vi "P1dB_Anritsu_SA.vi"(0 "VISA resource name":refnum<visa-resource-name>, 5 "Marker (10:Active Marker)":i32(ring)=10 items=["Marker 1", "Marker 2", "Marker 3", "Marker 4", "Marker 5", "Marker 6", "Marker 7", "Marker 8", "Marker 9", "Marker 10", "Active Marker"], 7 "Marker Type (0:Frequency or Time)":i32(ring) items=["Frequency or Time", "Level", "Position"], 11 "error in (no error)":errorcluster) -> (4 "VISA resource name out":refnum<visa-resource-name>, 6 "Marker_X Response":dbl format="%.3f", 10 "Marker_Y Response 2":dbl format="%.3f", 15 "error out":errorcluster)   [LabVIEW 2020]
doc: "Reads the active Marker data."
uses:
  Anritsu Signal Analyzer Series/Anritsu Signal Analyzer Series.lvlib
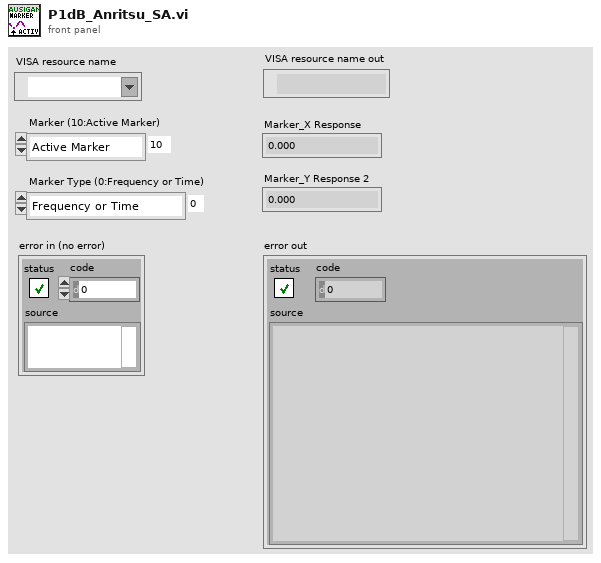
[diagram p1: front panel]
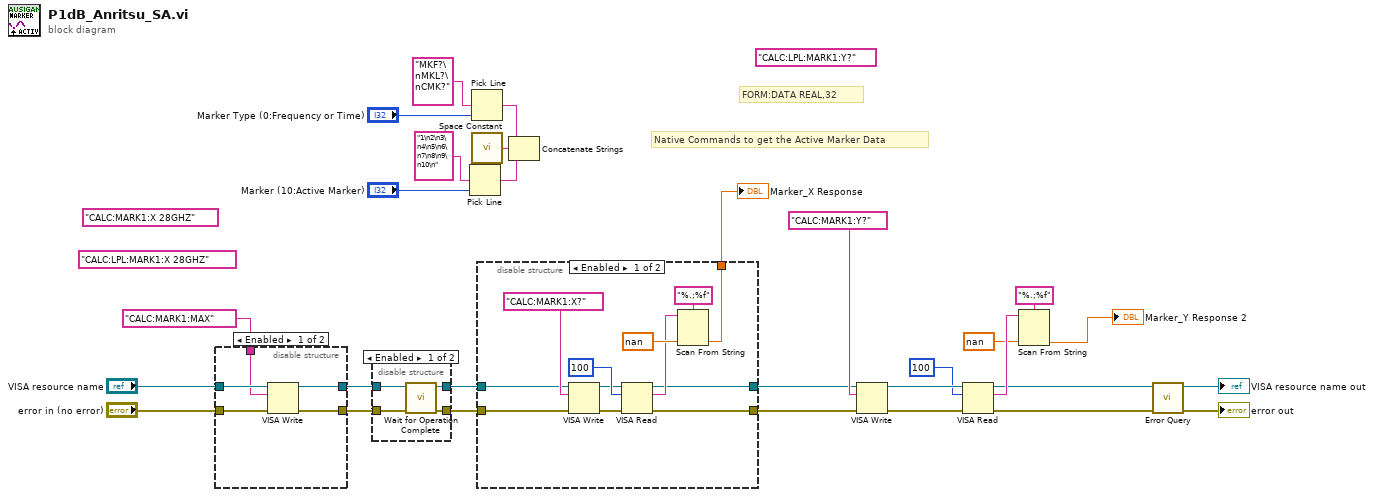
[diagram p0: block diagram]
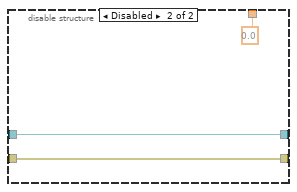
[diagram p2: hidden frame]
diagram:
  (unwired) "CALC:LPL:MARK1:Y?" ("write buffer")
  (unwired) "CALC:LPL:MARK1:X 28GHZ" ("write buffer")
  (unwired) "CALC:MARK1:X 28GHZ" ("write buffer")
  # "FORM:DATA REAL,32"
  # "Native Commands to get the Active Marker Data"
  n1 = disable-structure shown="Enabled" {
    disable-tunnel: "error in (no error)" -> [w34 w35]
    disable-tunnel: "VISA resource name" -> [w33 w36]
    disable-tunnel: [w32 w35] -> w17
    disable-tunnel: [w31 w36] -> w15
    disable-tunnel: "CALC:MARK1:MAX" ("write buffer") -> [w30 _]
    frame Enabled {
      n2 = VISA Write(VISA resource name=w33, write buffer=w30, error in (no error)=w34) -> (VISA resource name out=w31:refnum<visa-resource-name>, error out=w32:errorcluster)  [unwired: 1 out]
    }
    frame Disabled {
    }
  }
  n3 = disable-structure shown="Enabled" {
    disable-tunnel: w17 -> [w40 w41]
    disable-tunnel: [w39 w41] -> w16
    disable-tunnel: w15 -> [w38 w42]
    disable-tunnel: [w37 w42] -> w14
    frame Enabled {
      n4 = call "Wait for Operation Complete.vi"("error in (no error)"=w40, "VISA resource name"=w38) -> ("error out"=w39:errorcluster, "VISA resource name out"=w37:refnum<visa-resource-name>)  [unwired: 8 in]
    }
    frame Disabled {
    }
  }
  n5 = Pick Line(multi-line string="1\n2\n3\n4\n5\n6\n7\n8\n9\n10\n" ("文字列"), line index="Marker (10:Active Marker)") -> (output string=w24:string)  [unwired: 1 in]
  n6 = Pick Line(multi-line string="MKF?\nMKL?\nCMK?" ("_Command"), line index="Marker Type (0:Frequency or Time)") -> (output string=w20:string)  [unwired: 1 in]
  n7 = call <vilib>:"Space Constant.vi"() -> ("String"=w21:string)
  n8 = disable-structure shown="Enabled" {
    disable-tunnel: [w54 0.0 ("Marker_X Response")] -> w27
    disable-tunnel: w16 -> [w46 w56]
    disable-tunnel: w14 -> [w45 w57]
    disable-tunnel: [w44 w57] -> w2
    disable-tunnel: [w43 w56] -> w1
    frame Enabled {
      n9 = VISA Write(VISA resource name=w45, write buffer="CALC:MARK1:X?", error in (no error)=w46) -> (VISA resource name out=w48:refnum<visa-resource-name>, error out=w49:errorcluster)  [unwired: 1 out]
      n10 = VISA Read(VISA resource name=w48, byte count=u32 100 ("byte count (0)"), error in (no error)=w49) -> (VISA resource name out=w44:refnum<visa-resource-name>, read buffer=w51:string, error out=w43:errorcluster)  [unwired: 1 out]
      n11 = Scan From String(format string="%.;%f" ("Format String"), input string=w51, default 1=nan ("_Default")) -> (output 1=w54:dbl)  [unwired: 2 in, 3 out]
    }
    frame Disabled {
    }
  }
  "Marker_X Response" <- w27
  n12 = Concatenate Strings(w20, w21, w24) -> ()  [unwired: 1 out]
  n13 = VISA Write(VISA resource name=w2, write buffer="CALC:MARK1:Y?", error in (no error)=w1) -> (VISA resource name out=w12:refnum<visa-resource-name>, error out=w11:errorcluster)  [unwired: 1 out]
  n14 = VISA Read(VISA resource name=w12, byte count=u32 100 ("byte count (0)"), error in (no error)=w11) -> (VISA resource name out=w6:refnum<visa-resource-name>, read buffer=w9:string, error out=w5:errorcluster)  [unwired: 1 out]
  n15 = Scan From String(format string="%.;%f" ("Format String"), input string=w9, default 1=nan ("_Default")) -> (output 1=→"Marker_Y Response 2":dbl)  [unwired: 2 in, 3 out]
  n16 = call "Error Query.vi"("error in (no error)"=w5, "VISA resource name"=w6) -> ("error out"=→"error out":errorcluster, "VISA resource name out"=→"VISA resource name out":refnum<visa-resource-name>)  [unwired: 6 in, 2 out]
